vi "ATM.vi"() -> ()   [LabVIEW 2023]
panel:
  out "Ended":bool
  out "Decoration Indicator":bool
  out "Inserted":bool
  in  "End Button":bool
  in  "Decoration Button":bool
  in  "Insert Button":bool
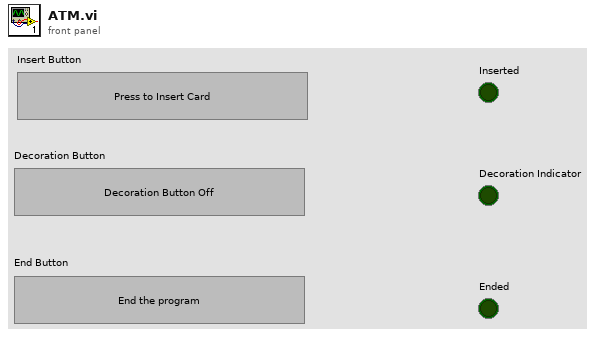
[diagram p1: front panel]
types:
  T1 = enum8{"Enabled", "Disabled", "Disabled and Grayed Out"}
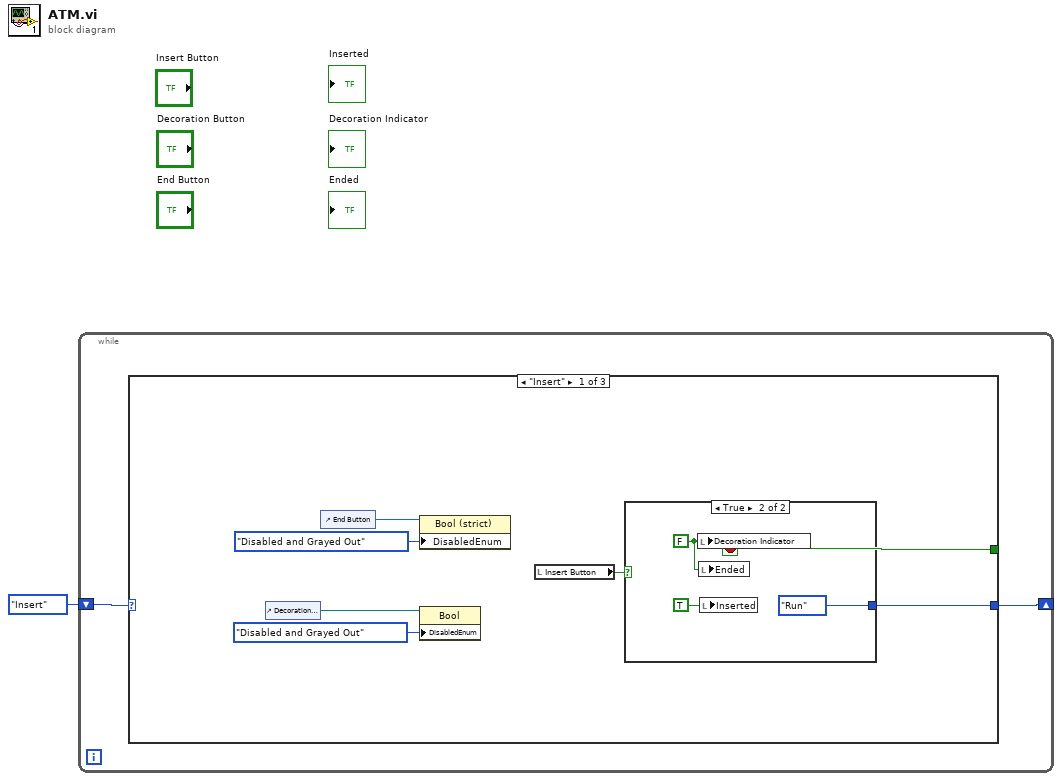
[diagram p0: block diagram]
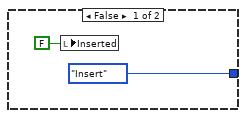
[diagram p2: hidden frame]
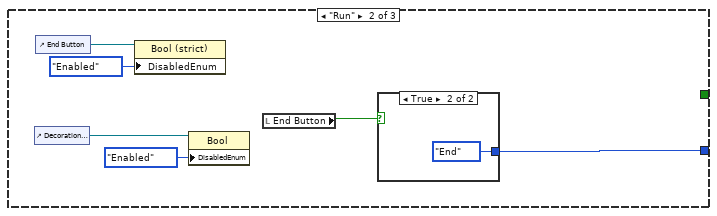
[diagram p3: hidden frame]
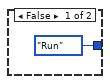
[diagram p4: hidden frame]
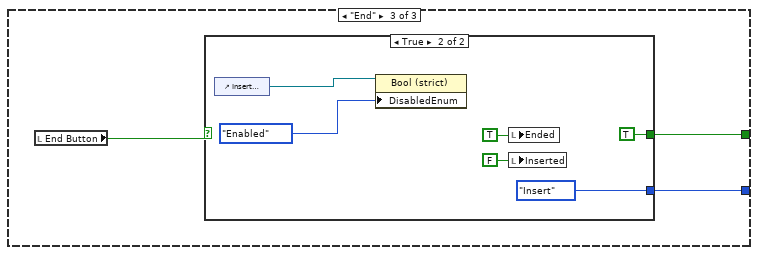
[diagram p5: hidden frame]
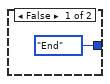
[diagram p6: hidden frame]
diagram:
  n1 = while {
    shift-right: [w3] -> _
    shift-left: enum16{"Insert", "Run", "End"}."Insert" -> [w4]
    stop <- w2 stop-if-true
    n2 = case shown="\"Insert\"" w4 {
      tunnel: [w9 w20 w25] -> w3
      tunnel: [_ _ w24] -> w2
      frame "Insert" {
        n3 = control-ref of="Decoration Button"() -> (w6:refnum<vi>)
        n4 = control-ref of="End Button"() -> (w8:refnum<vi>)
        n5 = property class="Bool (strict)"(reference=w8, "DisabledEnum"=T1."Disabled and Grayed Out" ("Disabled")) -> ()  [unwired: 1 in, 2 out]
        n6 = property class="Bool"(reference=w6, "DisabledEnum"=T1."Disabled and Grayed Out" ("Disabled")) -> ()  [unwired: 1 in, 2 out]
        n7 = local read "Insert Button"() -> (w10:bool)
        n8 = case shown="True" w10 {
          tunnel: [enum16{"Insert", "Run", "End"}."Insert" enum16{"Insert", "Run", "End"}."Run"] -> w9
          frame False {
            n9 = local write "Inserted"(FALSE) -> ()
          }
          frame True {
            w13 = FALSE ("Decoration Indicator")
            n10 = local write "Decoration Indicator"(w13) -> ()
            n11 = local write "Ended"(w13) -> ()
            n12 = local write "Inserted"(TRUE ("Inserted")) -> ()
          }
        }
      }
      frame "Run" {
        n13 = control-ref of="Decoration Button"() -> (w18:refnum<vi>)
        n14 = control-ref of="End Button"() -> (w19:refnum<vi>)
        n15 = property class="Bool (strict)"(reference=w19, "DisabledEnum"=T1."Enabled" ("Disabled")) -> ()  [unwired: 1 in, 2 out]
        n16 = property class="Bool"(reference=w18, "DisabledEnum"=T1."Enabled" ("Disabled")) -> ()  [unwired: 1 in, 2 out]
        n17 = local read "End Button"() -> (w21:bool)
        n18 = case shown="True" w21 {
          tunnel: [enum16{"Insert", "Run", "End"}."Run" enum16{"Insert", "Run", "End"}."End"] -> w20
          frame False {
          }
          frame True {
          }
        }
      }
      frame "End" {
        n19 = local read "End Button"() -> (w26:bool)
        n20 = case shown="True" w26 {
          tunnel: [enum16{"Insert", "Run", "End"}."End" enum16{"Insert", "Run", "End"}."Insert"] -> w25
          tunnel: [_ TRUE] -> w24
          frame False {
          }
          frame True {
            n21 = control-ref of="Insert Button"() -> (w29:refnum<vi>)
            n22 = property class="Bool (strict)"(reference=w29, "DisabledEnum"=T1."Enabled" ("Disabled")) -> ()  [unwired: 1 in, 2 out]
            n23 = local write "Ended"(TRUE ("Ended")) -> ()
            n24 = local write "Inserted"(FALSE ("Inserted")) -> ()
          }
        }
      }
    }
  }
